vi "rvc Create Revolute Link.vi"(6 "length (a)":dbl format="%#_13g", 7 "offset distance (d)":dbl, 8 "joint coordinate offset":dbl, 9 "twist angle (alpha)":dbl, 10 "rotation angle (theta)":dbl, 11 "Array 2":T1[](array[typedef])) -> (3 "Array":T1[](array[typedef]))   [LabVIEW 2014]
uses:
  <vilib>/robotics/Kinematics/DH Kinematic Parameters.ctl
  <vilib>/robotics/Kinematics/Link/Joint Type.ctl
  <vilib>/robotics/Kinematics/Link/NI_Robotics_Link.lvclass
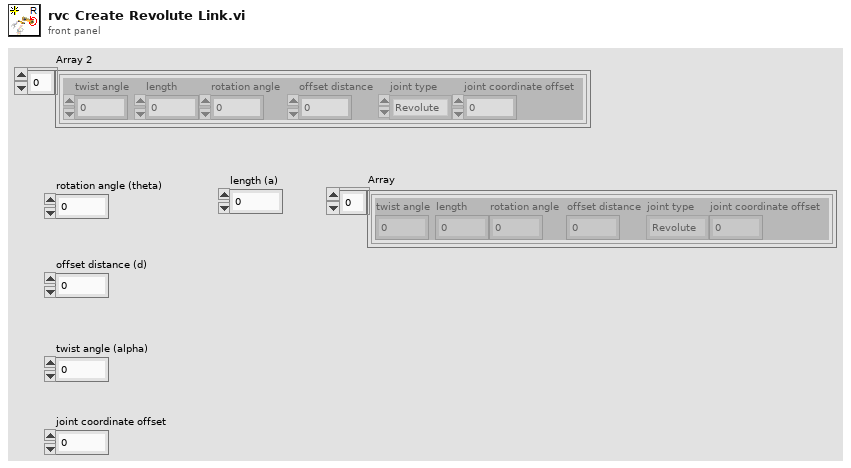
[diagram p1: front panel]
types:
  T1 = typedef "DH Kinematic Parameters.ctl" = cluster{"twist angle":dbl, "length":dbl, "rotation angle":dbl, "offset distance":dbl, "joint type":T2, "joint coordinate offset":dbl}
  T2 = typedef "NI_Robotics_Link.lvclass/Joint Type.ctl" = enum16{"Revolute", "Prismatic"}
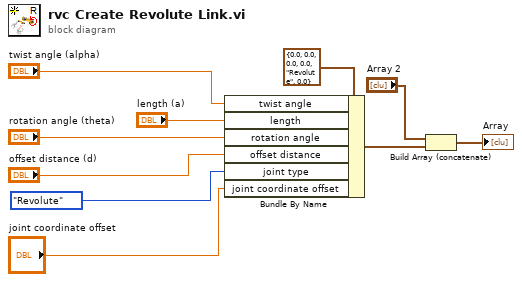
[diagram p0: block diagram]
diagram:
  n1 = Bundle By Name(cluster=T1 {"twist angle"=0.0, "length"=0.0, "rotation angle"=0.0, "offset distance"=0.0, "joint type"=enum."Revolute", "joint coordinate offset"=0.0} ("Link Parameters"), "twist angle"="twist angle (alpha)", "length"="length (a)", "rotation angle"="rotation angle (theta)", "offset distance"="offset distance (d)", "joint type"=Joint_Type."Revolute", "joint coordinate offset"="joint coordinate offset") -> (w2:T1)
  n2 = Build Array (concatenate)("Array 2", w2) -> (→"Array":T1[])
